vi "A2_Maquina_Estados01.vi"() -> ()   [LabVIEW 2025]
panel:
  out "Boolean 4":bool
  in  "stop":bool
  out "Boolean 3":bool
  out "Boolean 2":bool
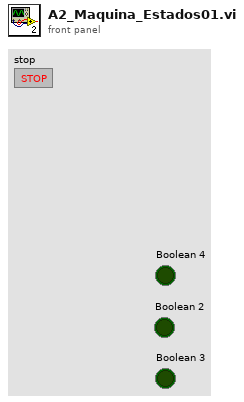
[diagram p1: front panel]
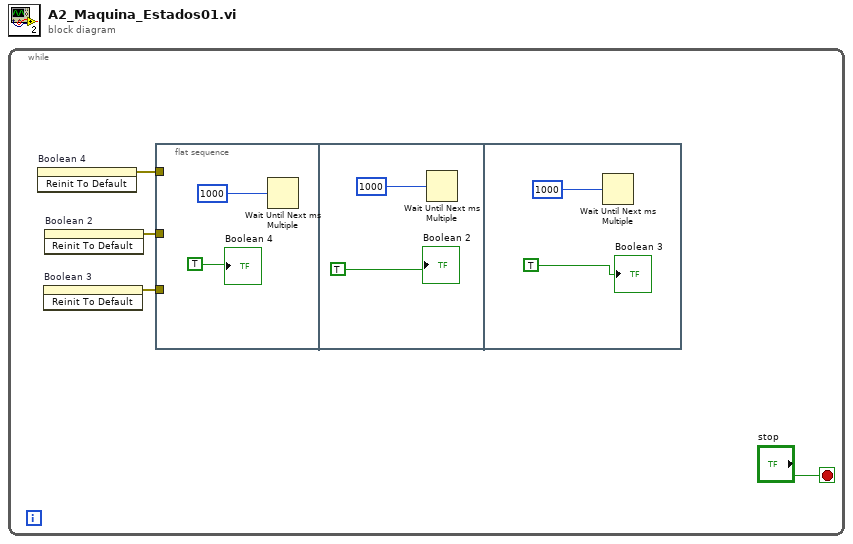
[diagram p0: block diagram]
diagram:
  n1 = while {
    stop <- "stop" stop-if-true
    n2 = invoke on="Boolean 4" class="Bool (strict)" method="Reinit To Default"() -> (error out=w1:errorcluster)  [unwired: 3 in, 2 out]
    n3 = invoke on="Boolean 3" class="Bool (strict)" method="Reinit To Default"() -> (error out=w2:errorcluster)  [unwired: 3 in, 2 out]
    n4 = invoke on="Boolean 2" class="Bool (strict)" method="Reinit To Default"() -> (error out=w3:errorcluster)  [unwired: 3 in, 2 out]
    n5 = flat-sequence {
      tunnel: w3 -> [_]
      tunnel: w2 -> [_]
      tunnel: w1 -> [_]
      frame #0 {
        n6 = Wait Until Next ms Multiple(millisecond multiple=u32 1000) -> ()  [unwired: 1 out]
        "Boolean 4" <- TRUE ("Boolean 2")
      }
      frame #1 {
        n7 = Wait Until Next ms Multiple(millisecond multiple=u32 1000) -> ()  [unwired: 1 out]
        "Boolean 2" <- TRUE ("Boolean 2")
      }
      frame #2 {
        n8 = Wait Until Next ms Multiple(millisecond multiple=u32 1000) -> ()  [unwired: 1 out]
        "Boolean 3" <- TRUE ("Boolean 2")
      }
    }
  }
